vi "CRYStepVIFilePath.vi"(7 "Category Name":string, 10 "Step Name":string) -> (0 "Run VI Path Out":path, 1 "FlattenVI path":path, 2 "Default StepFilePath":path, 3 "Editor VI Path Out":path, 4 "Special path":path)   [LabVIEW 2013]
uses:
  CRYMainGlobal.vi
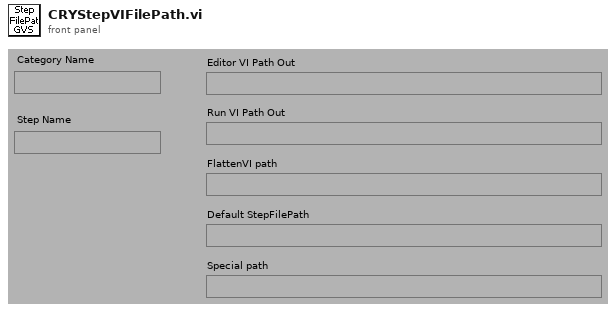
[diagram p1: front panel]
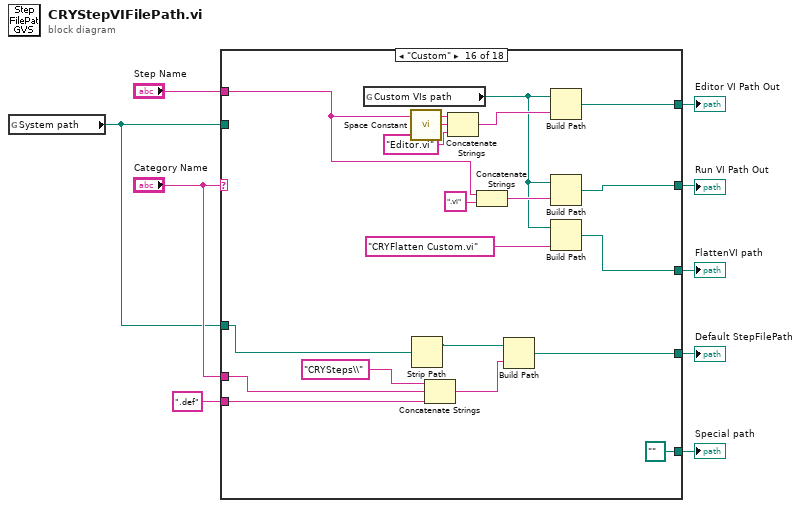
[diagram p0: block diagram]
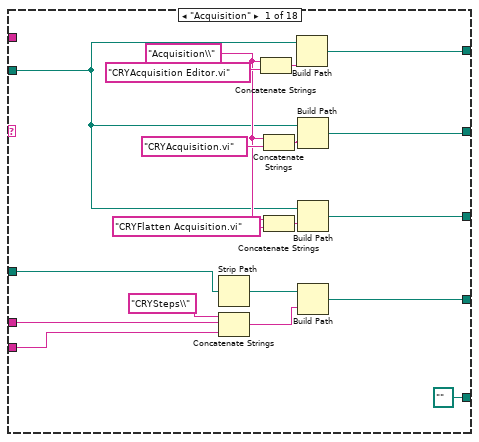
[diagram p2: hidden frame]
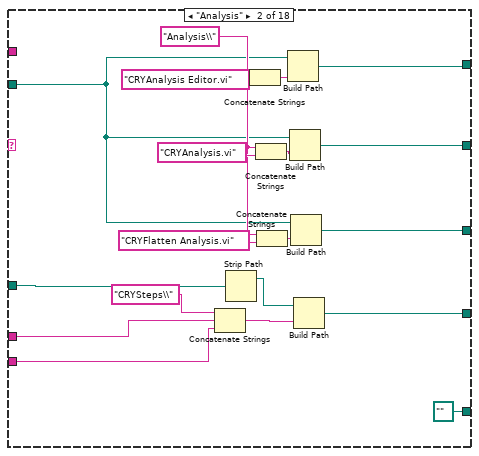
[diagram p3: hidden frame]
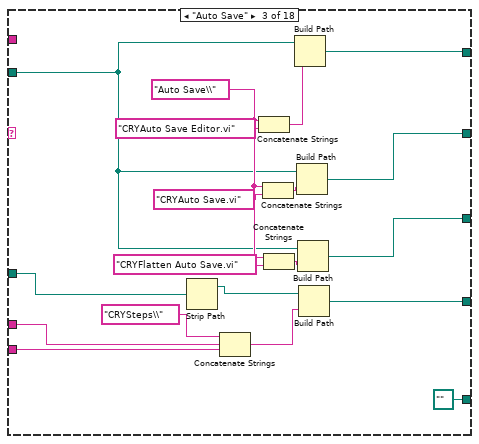
[diagram p4: hidden frame]
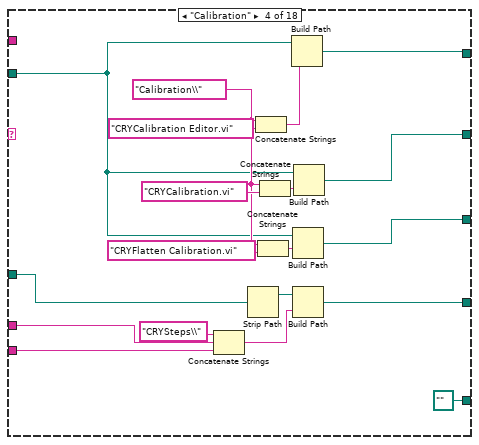
[diagram p5: hidden frame]
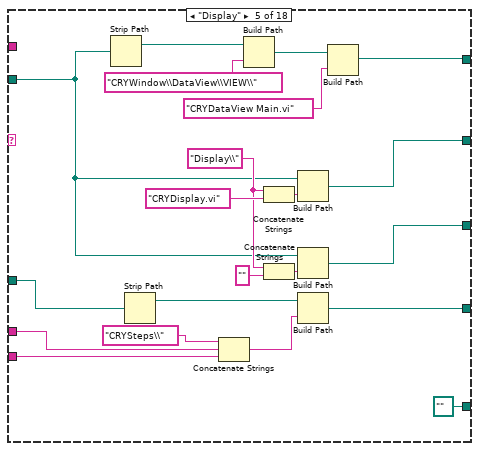
[diagram p6: hidden frame]
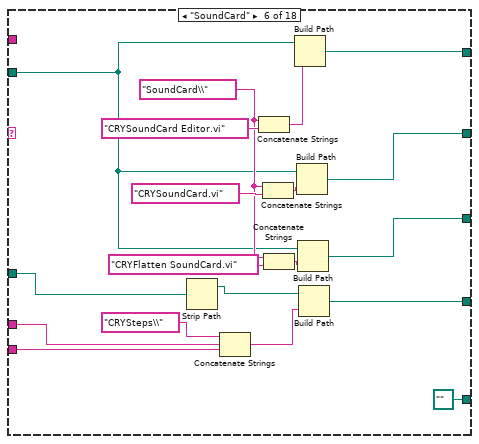
[diagram p7: hidden frame]
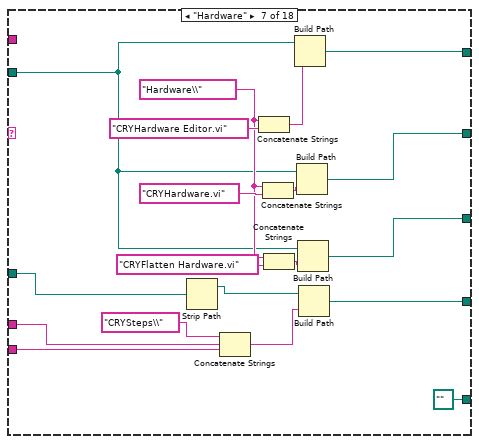
[diagram p8: hidden frame]
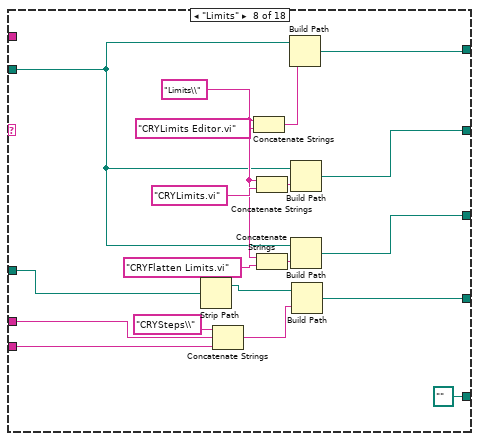
[diagram p9: hidden frame]
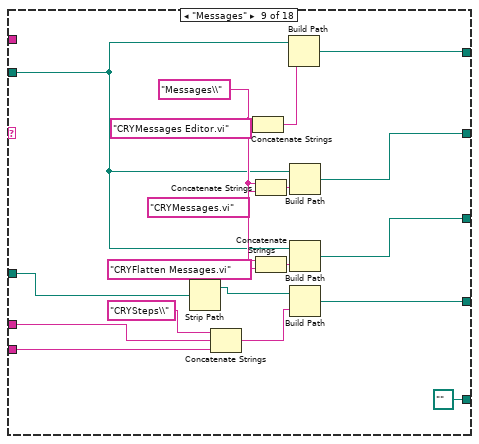
[diagram p10: hidden frame]
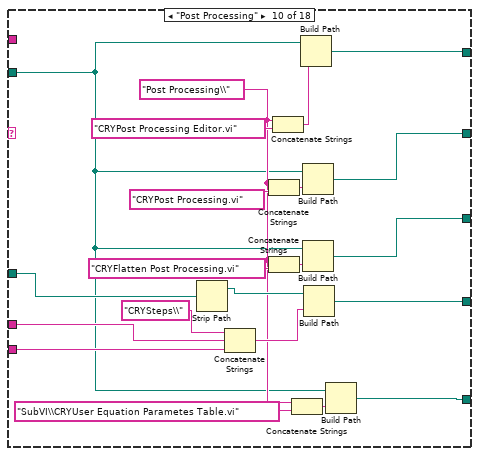
[diagram p11: hidden frame]
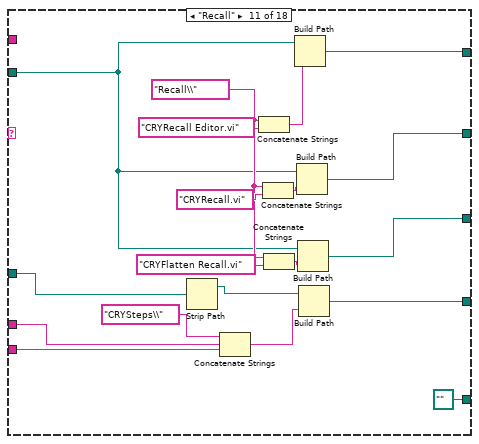
[diagram p12: hidden frame]
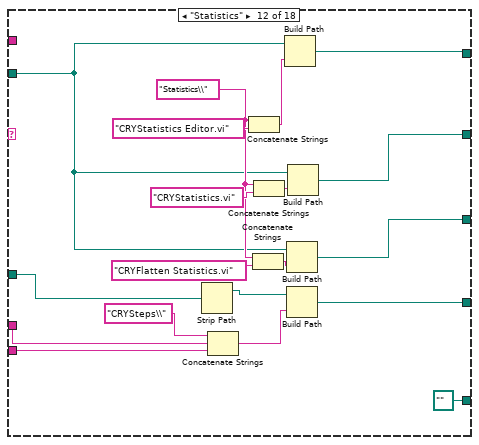
[diagram p13: hidden frame]
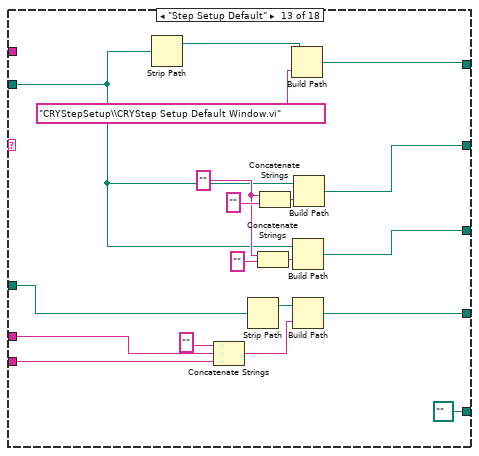
[diagram p14: hidden frame]
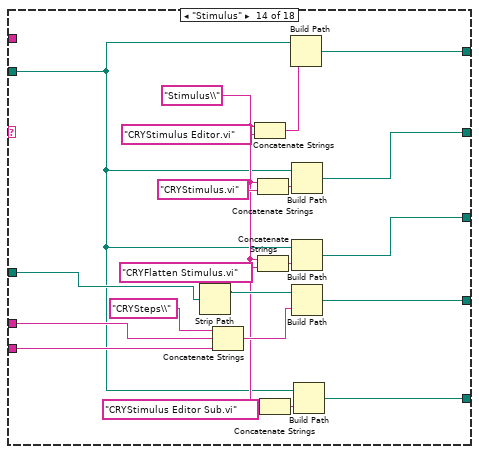
[diagram p15: hidden frame]
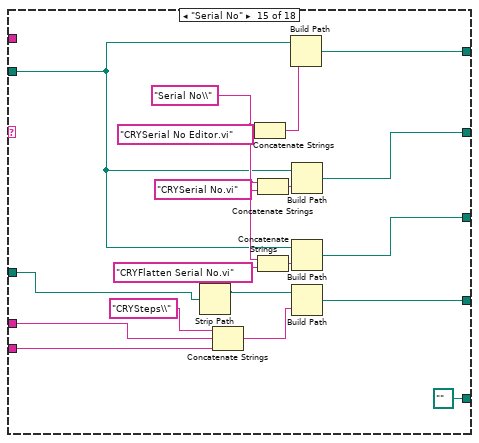
[diagram p16: hidden frame]
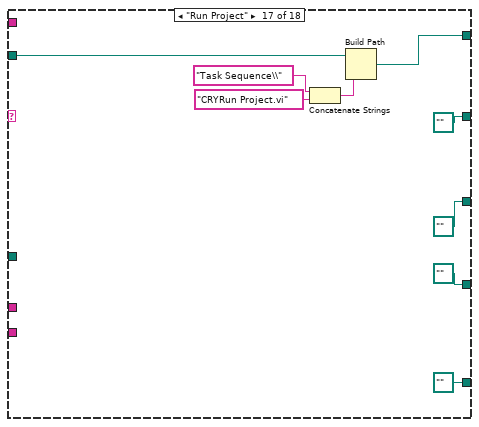
[diagram p17: hidden frame]
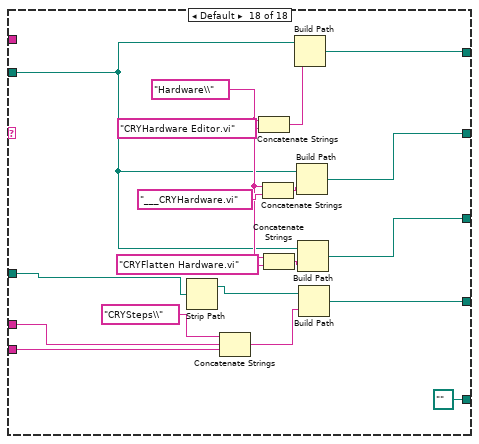
[diagram p18: hidden frame]
diagram:
  n1 = global read "CRYMainGlobal.vi" "System path"() -> (w2:path)
  n2 = case shown="\"Custom\"" "Category Name" {
    tunnel: w2 -> [w10 w29 w48 w67 w86 w107 w126 w145 w164 w183 w204 w223 w242 w261 w282 _ w320 w329]
    tunnel: [w26 w45 w64 w83 w106 w123 w142 w161 w180 w201 w220 w239 w260 w279 w298 w319 w321 w345] -> w9
    tunnel: [w23 w42 w61 w80 w89 w120 w139 w158 w177 w198 w217 w236 w257 w276 w295 w316 path "" ("appended path") w342] -> w8
    tunnel: [w19 w39 w58 w77 w102 w117 w136 w155 w174 w195 w214 w233 w254 w273 w292 w315 path "" ("appended path") w339] -> w7
    tunnel: "Category Name" -> [w18 w35 w54 w69 w99 w113 w132 w151 w170 w192 w210 w229 w251 w270 w289 w312 _ w335]
    tunnel: [w15 w34 w53 w73 w98 w112 w131 w150 w169 w191 w209 w228 w250 w269 w288 w311 path "" ("appended path") w334] -> w5
    tunnel: [path "" ("appended path") path "" ("appended path") path "" ("appended path") path "" ("appended path") path "" ("appended path") path "" ("appended path") path "" ("appended path") path "" ("appended path") path "" ("appended path") w185 path "" ("appended path") path "" ("appended path") path "" ("appended path") w265 path "" ("appended path") path "" ("appended path") path "" ("appended path") path "" ("appended path")] -> w4
    tunnel: ".def" ("string") -> [w12 w31 w50 w68 w95 w109 w128 w147 w166 w189 w206 w225 w247 w263 w285 w309 _ w331]
    tunnel: w2 -> [w11 w30 w49 w70 w87 w108 w127 w146 w165 w184 w205 w224 w243 w262 w283 w307 _ w330]
    tunnel: "Step Name" -> [_ _ _ _ _ _ _ _ _ _ _ _ _ _ _ w303 _ _]
    frame "Acquisition" {
      w20 = "Acquisition\\"
      n3 = Strip Path(path=w11) -> (stripped path=w14:path)  [unwired: 1 out]
      n4 = Concatenate Strings("CRYSteps\\" ("name or relative path"), w18, w12) -> (w16:string)
      n5 = Concatenate Strings(w20, "CRYAcquisition Editor.vi" ("string")) -> (w28:string)
      n6 = Concatenate Strings(w20, "CRYAcquisition.vi" ("string")) -> (w25:string)
      n7 = Concatenate Strings(w20, "CRYFlatten Acquisition.vi" ("string")) -> (w21:string)
      n8 = Build Path(base path=w10, name or relative path=w28) -> (appended path=w26:path)
      n9 = Build Path(base path=w10, name or relative path=w25) -> (appended path=w23:path)
      n10 = Build Path(base path=w10, name or relative path=w21) -> (appended path=w19:path)
      n11 = Build Path(base path=w14, name or relative path=w16) -> (appended path=w15:path)
    }
    frame "Analysis" {
      w38 = "Analysis\\"
      n12 = Concatenate Strings("CRYSteps\\" ("name or relative path"), w35, w31) -> (w36:string)
      n13 = Strip Path(path=w30) -> (stripped path=w33:path)  [unwired: 1 out]
      n14 = Concatenate Strings(w38, "CRYAnalysis Editor.vi" ("string")) -> (w47:string)
      n15 = Concatenate Strings(w38, "CRYAnalysis.vi" ("string")) -> (w44:string)
      n16 = Concatenate Strings(w38, "CRYFlatten Analysis.vi" ("string")) -> (w40:string)
      n17 = Build Path(base path=w29, name or relative path=w47) -> (appended path=w45:path)
      n18 = Build Path(base path=w29, name or relative path=w44) -> (appended path=w42:path)
      n19 = Build Path(base path=w29, name or relative path=w40) -> (appended path=w39:path)
      n20 = Build Path(base path=w33, name or relative path=w36) -> (appended path=w34:path)
    }
    frame "Auto Save" {
      w57 = "Auto Save\\"
      n21 = Strip Path(path=w49) -> (stripped path=w52:path)  [unwired: 1 out]
      n22 = Concatenate Strings("CRYSteps\\" ("name or relative path"), w54, w50) -> (w55:string)
      n23 = Concatenate Strings(w57, "CRYAuto Save Editor.vi" ("string")) -> (w66:string)
      n24 = Concatenate Strings(w57, "CRYAuto Save.vi" ("string")) -> (w63:string)
      n25 = Concatenate Strings(w57, "CRYFlatten Auto Save.vi" ("string")) -> (w59:string)
      n26 = Build Path(base path=w48, name or relative path=w66) -> (appended path=w64:path)
      n27 = Build Path(base path=w48, name or relative path=w63) -> (appended path=w61:path)
      n28 = Build Path(base path=w48, name or relative path=w59) -> (appended path=w58:path)
      n29 = Build Path(base path=w52, name or relative path=w55) -> (appended path=w53:path)
    }
    frame "Calibration" {
      w76 = "Calibration\\"
      n30 = Concatenate Strings("CRYSteps\\" ("name or relative path"), w69, w68) -> (w74:string)
      n31 = Strip Path(path=w70) -> (stripped path=w72:path)  [unwired: 1 out]
      n32 = Concatenate Strings(w76, "CRYCalibration Editor.vi" ("string")) -> (w85:string)
      n33 = Concatenate Strings(w76, "CRYFlatten Calibration.vi" ("string")) -> (w78:string)
      n34 = Concatenate Strings(w76, "CRYCalibration.vi" ("string")) -> (w82:string)
      n35 = Build Path(base path=w67, name or relative path=w85) -> (appended path=w83:path)
      n36 = Build Path(base path=w67, name or relative path=w78) -> (appended path=w77:path)
      n37 = Build Path(base path=w72, name or relative path=w74) -> (appended path=w73:path)
      n38 = Build Path(base path=w67, name or relative path=w82) -> (appended path=w80:path)
    }
    frame "Display" {
      w90 = "Display\\" ("string")
      n39 = Strip Path(path=w86) -> (stripped path=w88:path)  [unwired: 1 out]
      n40 = Strip Path(path=w87) -> (stripped path=w97:path)  [unwired: 1 out]
      n41 = Concatenate Strings("CRYSteps\\" ("name or relative path"), w99, w95) -> (w100:string)
      n42 = Build Path(base path=w88, name or relative path="CRYWindow\\DataView\\VIEW\\") -> (appended path=w92:path)
      n43 = Concatenate Strings(w90, "CRYDisplay.vi" ("string")) -> (w105:string)
      n44 = Concatenate Strings(w90, "" ("string")) -> (w103:string)
      n45 = Build Path(base path=w86, name or relative path=w105) -> (appended path=w89:path)
      n46 = Build Path(base path=w86, name or relative path=w103) -> (appended path=w102:path)
      n47 = Build Path(base path=w97, name or relative path=w100) -> (appended path=w98:path)
      n48 = Build Path(base path=w92, name or relative path="CRYDataView Main.vi" ("string")) -> (appended path=w106:path)
    }
    frame "SoundCard" {
      w116 = "SoundCard\\"
      n49 = Strip Path(path=w108) -> (stripped path=w111:path)  [unwired: 1 out]
      n50 = Concatenate Strings("CRYSteps\\" ("name or relative path"), w113, w109) -> (w114:string)
      n51 = Concatenate Strings(w116, "CRYSoundCard Editor.vi" ("string")) -> (w125:string)
      n52 = Concatenate Strings(w116, "CRYSoundCard.vi" ("string")) -> (w122:string)
      n53 = Concatenate Strings(w116, "CRYFlatten SoundCard.vi" ("string")) -> (w118:string)
      n54 = Build Path(base path=w107, name or relative path=w125) -> (appended path=w123:path)
      n55 = Build Path(base path=w107, name or relative path=w122) -> (appended path=w120:path)
      n56 = Build Path(base path=w107, name or relative path=w118) -> (appended path=w117:path)
      n57 = Build Path(base path=w111, name or relative path=w114) -> (appended path=w112:path)
    }
    frame "Hardware" {
      w135 = "Hardware\\"
      n58 = Strip Path(path=w127) -> (stripped path=w130:path)  [unwired: 1 out]
      n59 = Concatenate Strings("CRYSteps\\" ("name or relative path"), w132, w128) -> (w133:string)
      n60 = Concatenate Strings(w135, "CRYHardware Editor.vi" ("string")) -> (w144:string)
      n61 = Concatenate Strings(w135, "CRYHardware.vi" ("string")) -> (w141:string)
      n62 = Concatenate Strings(w135, "CRYFlatten Hardware.vi" ("string")) -> (w137:string)
      n63 = Build Path(base path=w126, name or relative path=w144) -> (appended path=w142:path)
      n64 = Build Path(base path=w126, name or relative path=w141) -> (appended path=w139:path)
      n65 = Build Path(base path=w126, name or relative path=w137) -> (appended path=w136:path)
      n66 = Build Path(base path=w130, name or relative path=w133) -> (appended path=w131:path)
    }
    frame "Limits" {
      w154 = "Limits\\"
      n67 = Strip Path(path=w146) -> (stripped path=w149:path)  [unwired: 1 out]
      n68 = Concatenate Strings("CRYSteps\\" ("name or relative path"), w151, w147) -> (w152:string)
      n69 = Concatenate Strings(w154, "CRYLimits Editor.vi" ("string")) -> (w163:string)
      n70 = Concatenate Strings(w154, "CRYLimits.vi" ("string")) -> (w160:string)
      n71 = Concatenate Strings(w154, "CRYFlatten Limits.vi" ("string")) -> (w156:string)
      n72 = Build Path(base path=w145, name or relative path=w163) -> (appended path=w161:path)
      n73 = Build Path(base path=w145, name or relative path=w160) -> (appended path=w158:path)
      n74 = Build Path(base path=w145, name or relative path=w156) -> (appended path=w155:path)
      n75 = Build Path(base path=w149, name or relative path=w152) -> (appended path=w150:path)
    }
    frame "Messages" {
      w173 = "Messages\\"
      n76 = Strip Path(path=w165) -> (stripped path=w168:path)  [unwired: 1 out]
      n77 = Concatenate Strings("CRYSteps\\" ("name or relative path"), w170, w166) -> (w171:string)
      n78 = Concatenate Strings(w173, "CRYMessages Editor.vi" ("string")) -> (w182:string)
      n79 = Concatenate Strings(w173, "CRYMessages.vi" ("string")) -> (w179:string)
      n80 = Concatenate Strings(w173, "CRYFlatten Messages.vi" ("string")) -> (w175:string)
      n81 = Build Path(base path=w164, name or relative path=w182) -> (appended path=w180:path)
      n82 = Build Path(base path=w164, name or relative path=w179) -> (appended path=w177:path)
      n83 = Build Path(base path=w164, name or relative path=w175) -> (appended path=w174:path)
      n84 = Build Path(base path=w168, name or relative path=w171) -> (appended path=w169:path)
    }
    frame "Post Processing" {
      w186 = "Post Processing\\"
      n85 = Strip Path(path=w184) -> (stripped path=w190:path)  [unwired: 1 out]
      n86 = Concatenate Strings("CRYSteps\\" ("name or relative path"), w192, w189) -> (w193:string)
      n87 = Concatenate Strings(w186, "CRYPost Processing.vi" ("string")) -> (w200:string)
      n88 = Concatenate Strings(w186, "CRYFlatten Post Processing.vi" ("string")) -> (w196:string)
      n89 = Concatenate Strings(w186, "CRYPost Processing Editor.vi" ("string")) -> (w203:string)
      n90 = Concatenate Strings(w186, "SubVI\\CRYUser Equation Parametes Table.vi" ("string")) -> (w187:string)
      n91 = Build Path(base path=w183, name or relative path=w203) -> (appended path=w201:path)
      n92 = Build Path(base path=w183, name or relative path=w200) -> (appended path=w198:path)
      n93 = Build Path(base path=w183, name or relative path=w196) -> (appended path=w195:path)
      n94 = Build Path(base path=w190, name or relative path=w193) -> (appended path=w191:path)
      n95 = Build Path(base path=w183, name or relative path=w187) -> (appended path=w185:path)
    }
    frame "Recall" {
      w213 = "Recall\\"
      n96 = Strip Path(path=w205) -> (stripped path=w208:path)  [unwired: 1 out]
      n97 = Concatenate Strings("CRYSteps\\" ("name or relative path"), w210, w206) -> (w211:string)
      n98 = Concatenate Strings(w213, "CRYRecall Editor.vi" ("string")) -> (w222:string)
      n99 = Concatenate Strings(w213, "CRYRecall.vi" ("string")) -> (w219:string)
      n100 = Concatenate Strings(w213, "CRYFlatten Recall.vi" ("string")) -> (w215:string)
      n101 = Build Path(base path=w204, name or relative path=w222) -> (appended path=w220:path)
      n102 = Build Path(base path=w204, name or relative path=w219) -> (appended path=w217:path)
      n103 = Build Path(base path=w204, name or relative path=w215) -> (appended path=w214:path)
      n104 = Build Path(base path=w208, name or relative path=w211) -> (appended path=w209:path)
    }
    frame "Statistics" {
      w232 = "Statistics\\"
      n105 = Strip Path(path=w224) -> (stripped path=w227:path)  [unwired: 1 out]
      n106 = Concatenate Strings("CRYSteps\\" ("name or relative path"), w229, w225) -> (w230:string)
      n107 = Concatenate Strings(w232, "CRYStatistics Editor.vi" ("string")) -> (w241:string)
      n108 = Concatenate Strings(w232, "CRYFlatten Statistics.vi" ("string")) -> (w234:string)
      n109 = Concatenate Strings(w232, "CRYStatistics.vi" ("string")) -> (w238:string)
      n110 = Build Path(base path=w223, name or relative path=w241) -> (appended path=w239:path)
      n111 = Build Path(base path=w223, name or relative path=w234) -> (appended path=w233:path)
      n112 = Build Path(base path=w227, name or relative path=w230) -> (appended path=w228:path)
      n113 = Build Path(base path=w223, name or relative path=w238) -> (appended path=w236:path)
    }
    frame "Step Setup Default" {
      w246 = "" ("string")
      n114 = Strip Path(path=w242) -> (stripped path=w244:path)  [unwired: 1 out]
      n115 = Concatenate Strings("" ("name or relative path"), w251, w247) -> (w252:string)
      n116 = Strip Path(path=w243) -> (stripped path=w249:path)  [unwired: 1 out]
      n117 = Concatenate Strings(w246, "" ("string")) -> (w255:string)
      n118 = Concatenate Strings(w246, "" ("string")) -> (w259:string)
      n119 = Build Path(base path=w244, name or relative path="CRYStepSetup\\CRYStep Setup Default Window.vi" ("string")) -> (appended path=w260:path)
      n120 = Build Path(base path=w242, name or relative path=w255) -> (appended path=w254:path)
      n121 = Build Path(base path=w249, name or relative path=w252) -> (appended path=w250:path)
      n122 = Build Path(base path=w242, name or relative path=w259) -> (appended path=w257:path)
    }
    frame "Stimulus" {
      w264 = "Stimulus\\"
      n123 = Strip Path(path=w262) -> (stripped path=w268:path)  [unwired: 1 out]
      n124 = Concatenate Strings("CRYSteps\\" ("name or relative path"), w270, w263) -> (w271:string)
      n125 = Concatenate Strings(w264, "CRYStimulus Editor.vi" ("string")) -> (w281:string)
      n126 = Concatenate Strings(w264, "CRYStimulus.vi" ("string")) -> (w278:string)
      n127 = Concatenate Strings(w264, "CRYFlatten Stimulus.vi" ("string")) -> (w274:string)
      n128 = Concatenate Strings(w264, "CRYStimulus Editor Sub.vi" ("string")) -> (w266:string)
      n129 = Build Path(base path=w261, name or relative path=w281) -> (appended path=w279:path)
      n130 = Build Path(base path=w261, name or relative path=w278) -> (appended path=w276:path)
      n131 = Build Path(base path=w261, name or relative path=w274) -> (appended path=w273:path)
      n132 = Build Path(base path=w268, name or relative path=w271) -> (appended path=w269:path)
      n133 = Build Path(base path=w261, name or relative path=w266) -> (appended path=w265:path)
    }
    frame "Serial No" {
      w286 = "Serial No\\"
      n134 = Strip Path(path=w283) -> (stripped path=w287:path)  [unwired: 1 out]
      n135 = Concatenate Strings("CRYSteps\\" ("name or relative path"), w289, w285) -> (w290:string)
      n136 = Concatenate Strings(w286, "CRYSerial No Editor.vi" ("string")) -> (w300:string)
      n137 = Concatenate Strings(w286, "CRYSerial No.vi" ("string")) -> (w297:string)
      n138 = Concatenate Strings(w286, "CRYFlatten Serial No.vi" ("string")) -> (w293:string)
      n139 = Build Path(base path=w282, name or relative path=w300) -> (appended path=w298:path)
      n140 = Build Path(base path=w282, name or relative path=w297) -> (appended path=w295:path)
      n141 = Build Path(base path=w282, name or relative path=w293) -> (appended path=w292:path)
      n142 = Build Path(base path=w287, name or relative path=w290) -> (appended path=w288:path)
    }
    frame "Custom" {
      n143 = global read "CRYMainGlobal.vi" "Custom VIs path"() -> (w301:path)
      n144 = call <vilib>:"Space Constant.vi"() -> ("String"=w305:string)
      n145 = Strip Path(path=w307) -> (stripped path=w310:path)  [unwired: 1 out]
      n146 = Concatenate Strings("CRYSteps\\" ("name or relative path"), w312, w309) -> (w313:string)
      n147 = Concatenate Strings(w303, w305, "Editor.vi" ("string")) -> (w304:string)
      n148 = Concatenate Strings(w303, ".vi" ("string")) -> (w318:string)
      n149 = Build Path(base path=w310, name or relative path=w313) -> (appended path=w311:path)
      n150 = Build Path(base path=w301, name or relative path=w304) -> (appended path=w319:path)
      n151 = Build Path(base path=w301, name or relative path=w318) -> (appended path=w316:path)
      n152 = Build Path(base path=w301, name or relative path="CRYFlatten Custom.vi" ("string")) -> (appended path=w315:path)
    }
    frame "Run Project" {
      n153 = Concatenate Strings("Task Sequence\\", "CRYRun Project.vi" ("string")) -> (w324:string)
      n154 = Build Path(base path=w320, name or relative path=w324) -> (appended path=w321:path)
    }
    frame Default {
      w338 = "Hardware\\"
      n155 = Strip Path(path=w330) -> (stripped path=w333:path)  [unwired: 1 out]
      n156 = Concatenate Strings("CRYSteps\\" ("name or relative path"), w335, w331) -> (w336:string)
      n157 = Concatenate Strings(w338, "CRYHardware Editor.vi" ("string")) -> (w347:string)
      n158 = Concatenate Strings(w338, "___CRYHardware.vi" ("string")) -> (w344:string)
      n159 = Concatenate Strings(w338, "CRYFlatten Hardware.vi" ("string")) -> (w340:string)
      n160 = Build Path(base path=w329, name or relative path=w347) -> (appended path=w345:path)
      n161 = Build Path(base path=w329, name or relative path=w344) -> (appended path=w342:path)
      n162 = Build Path(base path=w329, name or relative path=w340) -> (appended path=w339:path)
      n163 = Build Path(base path=w333, name or relative path=w336) -> (appended path=w334:path)
    }
  }
  "Editor VI Path Out" <- w9
  "Run VI Path Out" <- w8
  "FlattenVI path" <- w7
  "Default StepFilePath" <- w5
  "Special path" <- w4
